vi "Get pos axis.vi"(8 "error in (no error)":errorcluster, 10 "Axis":i32=1 min=1 max=4, 11 "DelayLineLS4 in":refnum<class "DLLS4.lvclass">) -> (0 "error out":errorcluster, 2 "Pos":dbl, 3 "DelayLineLS4 out":refnum<class "DLLS4.lvclass">)   [LabVIEW 2020, in "DLLS4.lvclass"]
uses:
  DLLS4.lvclass
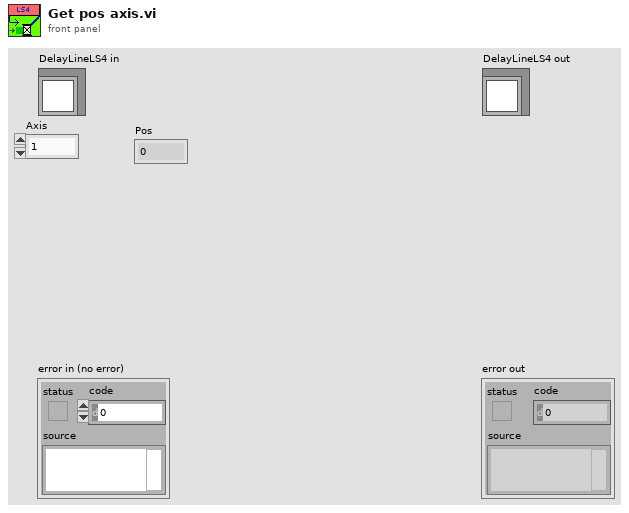
[diagram p1: front panel]
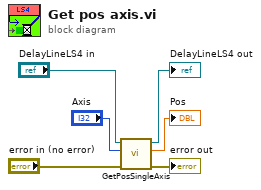
[diagram p0: block diagram]
diagram:
  n1 = call-dynamic "GetPosSingleAxis.vi"("error in (no error)"="error in (no error)", "Axis"="Axis", "DelayLineLS4 en entrée"="DelayLineLS4 in") -> ("error out"=→"error out":errorcluster, "Pos"=→"Pos":dbl, "DelayLineLS4 en sortie"=→"DelayLineLS4 out":refnum<class "DLLS4.lvclass">)  [unwired: 6 in]
